vi "get_ports.vi"(5 "error in (no error)":errorcluster, 6 "VISA Refnum in":refnum<visa-resource-name>) -> (0 "error out":errorcluster, 1 "VISA Refnum out":refnum<visa-resource-name>, 2 "P1":T1, 3 "P0":T2, 4 "data":u8)   [LabVIEW 2014]
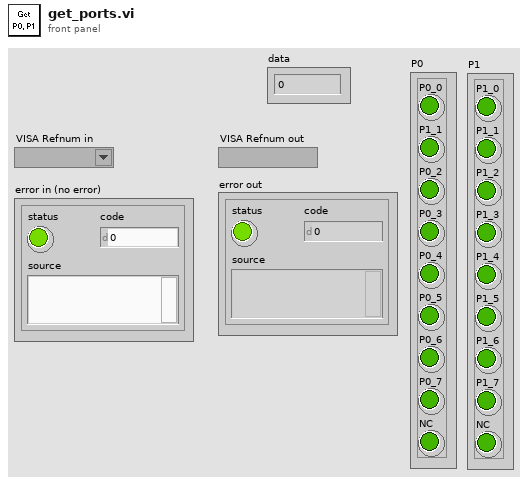
[diagram p1: front panel]
types:
  T1 = cluster{"P1_0":bool, "P1_1":bool, "P1_2":bool, "P1_3":bool, "P1_4":bool, "P1_5":bool, "P1_6":bool, "P1_7":bool, "NC":bool}
  T2 = cluster{"P0_0":bool, "P1_1":bool, "P0_2":bool, "P0_3":bool, "P0_4":bool, "P0_5":bool, "P0_6":bool, "P0_7":bool, "NC":bool}
  T3 = cluster{"Boolean array[0]":bool, "Boolean array[1]":bool, "Boolean array[2]":bool, "Boolean array[3]":bool, "Boolean array[4]":bool, "Boolean array[5]":bool, "Boolean array[6]":bool, "Boolean array[7]":bool, "Boolean array[8]":bool}
  T4 = cluster{"Boolean array[2]":bool, "Boolean array[4]":bool, "Boolean array[6]":bool, "Boolean array[0]":bool, "Boolean array[3]":bool, "Boolean array[5]":bool, "Boolean array[7]":bool, "Boolean array[1]":bool}
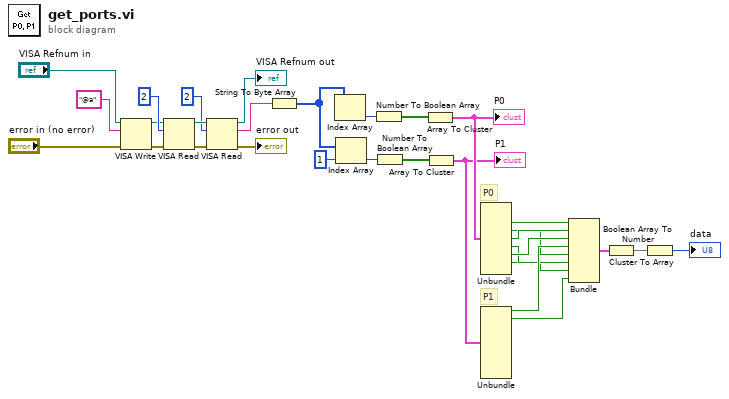
[diagram p0: block diagram]
diagram:
  # "P1"
  # "P0"
  n1 = VISA Write(VISA resource name="VISA Refnum in", write buffer="@a", error in (no error)="error in (no error)") -> (VISA resource name out=w28:refnum<visa-resource-name>, error out=w29:errorcluster)  [unwired: 1 out]
  n2 = VISA Read(VISA resource name=w28, byte count=u32 2, error in (no error)=w29) -> (VISA resource name out=w21:refnum<visa-resource-name>, error out=w22:errorcluster)  [unwired: 2 out]
  n3 = VISA Read(VISA resource name=w21, byte count=u32 2, error in (no error)=w22) -> (VISA resource name out=→"VISA Refnum out":refnum<visa-resource-name>, read buffer=w25:string, error out=→"error out":errorcluster)  [unwired: 1 out]
  n4 = String To Byte Array(string=w25) -> (unsigned byte array=w17:u8[])
  n5 = Index Array(array=w17) -> (element=w19:u8)  [unwired: 1 in]
  n6 = Index Array(array=w17, index=1) -> (element=w18:u8)
  n7 = Number To Boolean Array(number=w19) -> (Boolean array=w15:bool[])
  n8 = Number To Boolean Array(number=w18) -> (Boolean array=w14:bool[])
  n9 = Array To Cluster(array=w15) -> (cluster=w12:T3)
  "P0" <- w12
  n10 = Array To Cluster(array=w14) -> (cluster=w8:T3)
  "P1" <- w8
  n11 = Unbundle(w12) -> ("Boolean array[2]"=w13:bool, "Boolean array[3]"=w7:bool, "Boolean array[4]"=w11:bool, "Boolean array[5]"=w6:bool, "Boolean array[6]"=w10:bool, "Boolean array[7]"=w5:bool)  [unwired: 3 out]
  n12 = Unbundle(w8) -> ("Boolean array[0]"=w9:bool, "Boolean array[1]"=w4:bool)  [unwired: 7 out]
  n13 = Bundle("Boolean array[2]"=w13, "Boolean array[4]"=w11, "Boolean array[6]"=w10, "Boolean array[0]"=w9, "Boolean array[3]"=w7, "Boolean array[5]"=w6, "Boolean array[7]"=w5, "Boolean array[1]"=w4) -> (w3:T4)  [unwired: 1 in]
  n14 = Cluster To Array(cluster=w3) -> (array=w2:bool[])
  n15 = Boolean Array To Number(Boolean array=w2) -> (number=→"data":u32)
